vi "SendData.vi"(10 "Enum":enum16{"Add", "Take"}(ring), 11 "Spectras-Analiza":cluster{dbl[], dbl[]}[](array[cluster])) -> (2 "Spectras-Analiza 2":cluster{dbl[], dbl[]}[](array[cluster]))   [LabVIEW 2020]
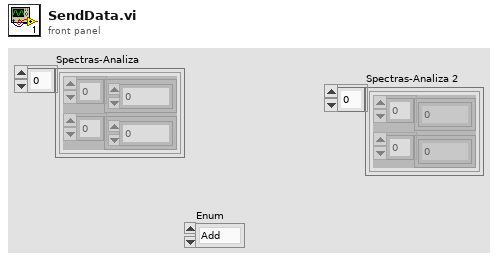
[diagram p1: front panel]
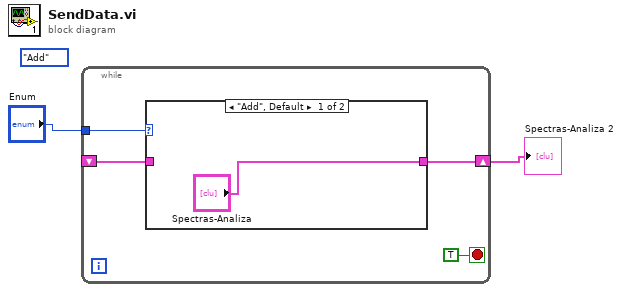
[diagram p0: block diagram]
diagram:
  (unwired) enum16{"Add", "Take"}."Add"
  n1 = while {
    shift-right: [w5] -> w1
    shift-left: _ -> [w3]
    tunnel: "Enum" -> [w4]
    stop <- TRUE stop-if-true
    n2 = case shown="\"Add\", Default" w4 {
      tunnel: ["Spectras-Analiza" w8] -> w5
      tunnel: w3 -> [_ w8]
      frame "Add", Default {
      }
      frame "Take" {
      }
    }
  }
  "Spectras-Analiza 2" <- w1
